vi "Dashboard Main.vi"() -> ()   [LabVIEW 2013]
uses:
  Vision/TargetType.ctl
  <vilib>/event_ctls.llb/eventvkey.ctl
  <vilib>/Rock Robotics/WPI/Dashboard/WPI_DashboardLogging Global.vi
  <vilib>/Utility/config.llb/Write Key (String).vi
  <vilib>/Utility/config.llb/Write Key (I32).vi
  <vilib>/Utility/config.llb/NI_LVConfig.lvlib
panel:
  out "Image Message":string="Timeout in Camera Communications"
  in  "Rec Mode":enum32{"Stop", "Record", "Playback"}(radio)
  in  "Dashboard Tab":T1(tab)
  in  "Camera Settings":T2={"Frame Rate"=30, "Compression"=30, "Size"=1} {"Frame Rate" scale=1.0..30.0; "Size" items=["640x480", "320x240", "160x120"]}
  out "MotorSliders R":cluster{"MotorSlide1":dbl, "MotorSlide2":dbl} {"MotorSlide2" scale=-1.0..1.0 scale format="%#_2e"; "MotorSlide1" scale=-1.0..1.0 scale format="%#_2e"}
  out "MotorChart R":cluster{"Numeric":dbl, "Numeric":dbl}(graph)
  out "MotorSliders L":T3 {"MotorSlide4 2" scale=0.0..14.0 scale format="%#_2e"; "MotorSlide2" scale=-1.0..1.0 scale format="%#_2e"; "MotorSlide1" scale=-1.0..1.0 scale format="%#_2e"}
  out "MotorChart L":T4(graph)
  out "JS1 Z":dbl(slide) scale=-1.0..1.0 scale format="%#_2e"
  out "Joystick 1":cluster{"X":dbl, "Y":dbl}[](graph)
  out "JS Buttons 1":T5
  out "JS2 Z":dbl(slide) scale=-1.0..1.0 scale format="%#_2e"
  out "Joystick 2":cluster{"X":dbl, "Y":dbl}[](graph)
  out "JS Buttons 2":T5
  out "Mode":T6(ring)=enum."Auto Disabled"
  out "Camera IP":string
  in  "DB Camera Config":bool
  out "fps":dbl format="%#.1g"
  out "Mbps":dbl format="%#.1g"
  out "Mbps 2":bool
  out "LED 1":bool
  in  "Color Components":T7={"Hue"={110.0, 142.0}, "Sat"={138.0, 255.0}, "Val"={139.0, 198.0}} {"Val" scale=0.0..255.0; "Sat" scale=0.0..255.0; "Hue" scale=0.0..255.0 scale format="%#_3g"}
  out "Distances":T9(array[cluster])
  in  "Test Slider":dbl(slide) scale=0.0..100.0 scale format="%#_3g"
  in  "On/Off":bool caption="Solenoid"
  in  "Test Name":u16(ring) items=["Select the test to run...", "Example Test", "-------------------------------", "List of tests is built in robot code.", "Replace with your own automated tests."]
  in  "Test Tree":string(tree)
  in  "Motor":cluster{"Value":dbl, "Enable":bool} {"Value" scale=-1.0..1.0 scale format="%#_3g"}
  out "Progress":T10 {"Test Progress" scale=0.0..100.0}
  in  "Rev/Fwd":cluster{"Forward":bool, "Reverse":bool}
  in  "Test Ring":u16(ring) items=["Auto", "Fixed indoor", "Fixed outdoor 1", "Fixed outdoor 2", "Fixed fluorescent 1", "Fixed fluorescent 2", "Hold current"]
  in  "Listbox":i32(listbox)
  out "Tree":string(tree)
  out "Camera Image":T11(plugin-control)
  in  "Enable":bool
  # "Left"
  # "Front"
  # "Right"
  # "Battery"
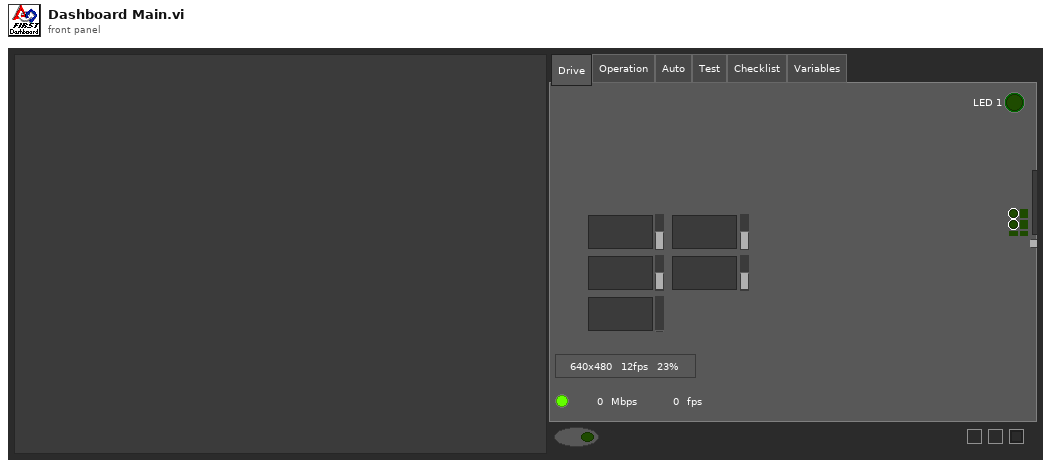
[diagram p1: front panel]
types:
  T1 = enum32{"Drive", "Operation", "Auto", "Test", "Checklist", "Variables"}
  T2 = cluster{"Frame Rate":i32, "Compression":i32, "Size":u16}
  T3 = cluster{"MotorSlide1":dbl, "MotorSlide2":dbl, "MotorSlide4 2":dbl}
  T4 = cluster{"Numeric":dbl, "Numeric":dbl, "Battery":sgl}
  T5 = cluster{bool, bool, bool, bool, bool, bool, bool, bool, bool, bool, bool, bool}
  T6 = enum8{"Tele-Op Disabled", "Tele-Op Enabled", "Auto Disabled", "Auto Enabled", "Test Disabled", "Test Enabled", ""}
  T7 = cluster{"Hue":cluster{dbl, dbl}, "Sat":cluster{dbl, dbl}, "Val":cluster{dbl, dbl}}
  T8 = typedef "TargetType.ctl" = enum16{"Not Hot", "Hot"}
  T9 = cluster{"Distance (ft)":dbl, "Target Center (-1 to 1)":cluster{"X":dbl, "Y":dbl}, "Left":bool, "State":T8}[]
  T10 = cluster{"Test Progress":u8, "Test Progress Text":string}
  T11 = typedef "IMAQ Image.ctl" = refnum<image>
  T12 = typedef "Image Type" = u32
  T13 = cluster{cluster{dbl, dbl}, cluster{dbl, dbl}, cluster{dbl, dbl}}
  T14 = cluster{"Digital Inputs":bool[], "Digital Outputs":bool[]}
  T15 = cluster{"Competition mode":bool, "Robot Link":bool, "Autonomous":bool, "Enabled":bool, "E-Stop":bool, "Simulated":bool, "TestMode":bool, "Docked Window":bool}
  T16 = typedef "NI_LVConfig.lvlib/Config Data RefNum.ctl" = refnum<k1>
  T17 = typedef "eventvkey.ctl" = enum16{"ASCII", "Enter", "Return", "Shift", "Ctrl", "Alt", "Cmd", "Opt", "Caps", "NumLock", "Clear", "Break", "Up", "Down", "Left", "Right", "Insert", "Delete", "Home", "End", "PageUp", "PageDown", "Escape", "Help", "Pause", "ScrollLock", "F1", "F2", "F3", "F4", "F5", "F6", "F7", "F8", "F9", "F10", "F11", "F12", "F13", "F14", "F15", "F16", "F17", "F18", "F19", "F20", "F21", "F22", "F23", "F24", "Play", "VolumeUp", "VolumeDown", "Mute", "Two Byte Char"}
  T18 = cluster{"Image Size":bool, "Image Type":bool, "Pixel Value":bool, "ROI Information":bool, "Zoom Factor":bool}
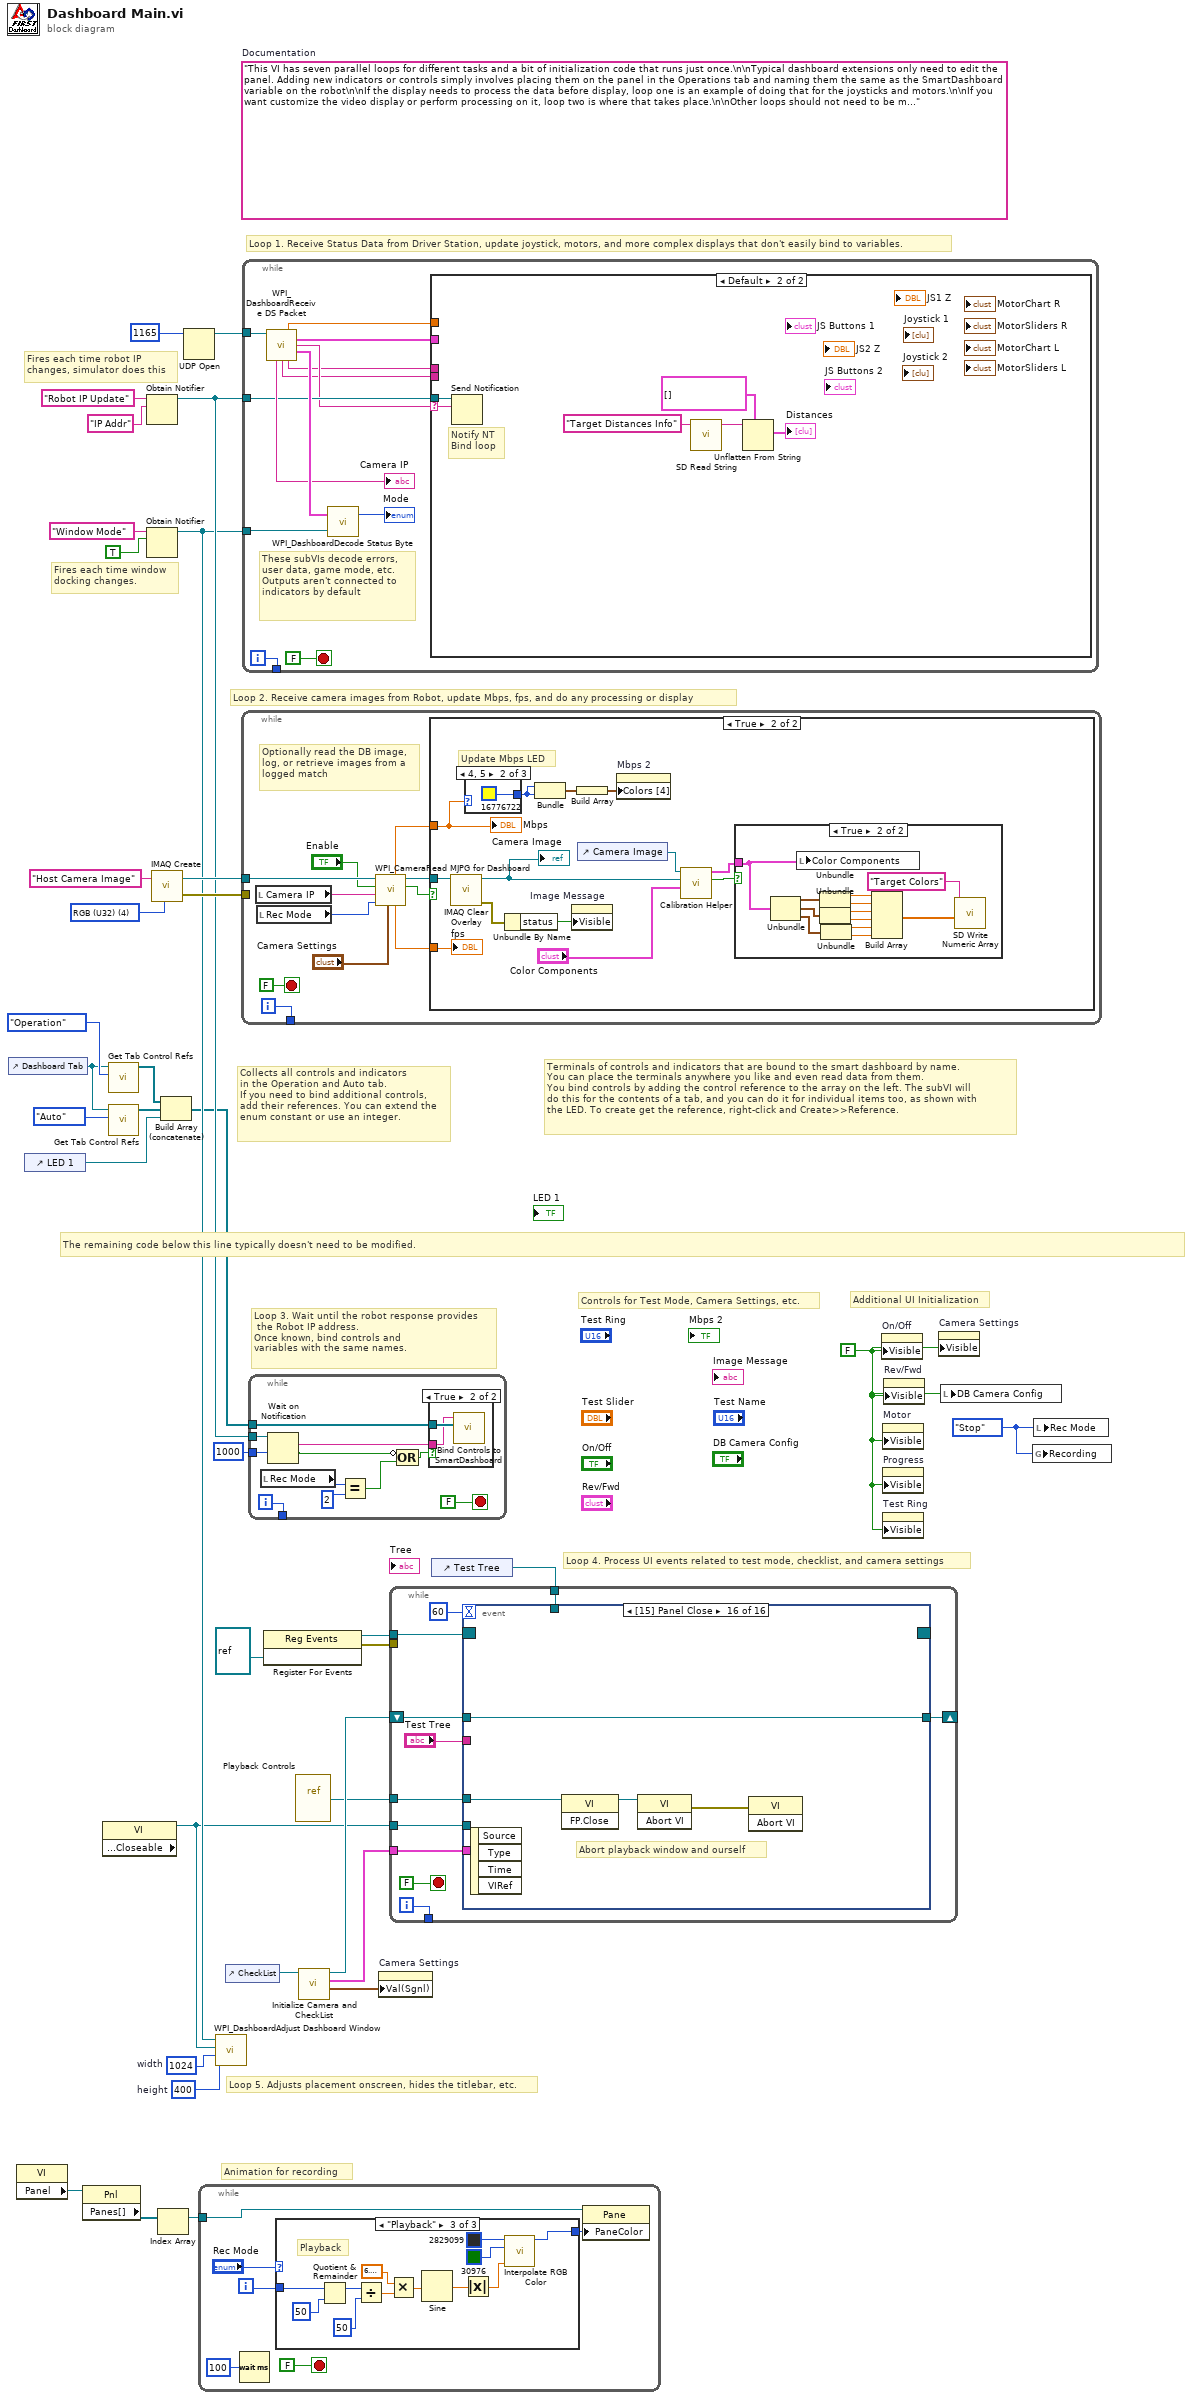
[diagram p0: block diagram]
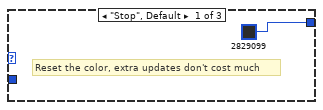
[diagram p2: hidden frame]
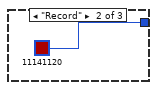
[diagram p3: hidden frame]
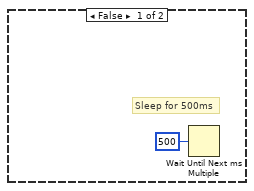
[diagram p5: hidden frame]
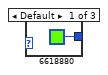
[diagram p7: hidden frame]
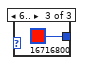
[diagram p8: hidden frame]
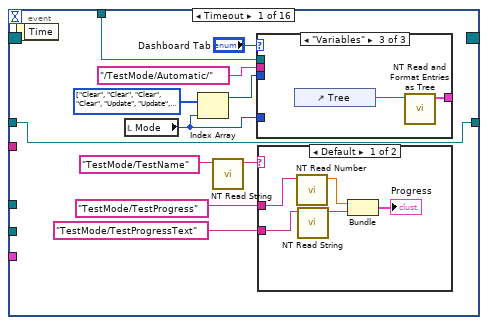
[diagram p9: hidden frame]
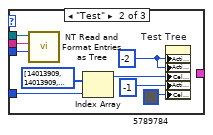
[diagram p11: hidden frame]
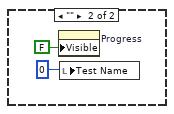
[diagram p12: hidden frame]
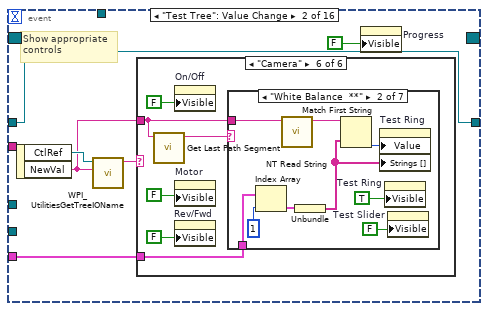
[diagram p13: hidden frame]
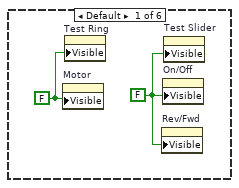
[diagram p14: hidden frame]
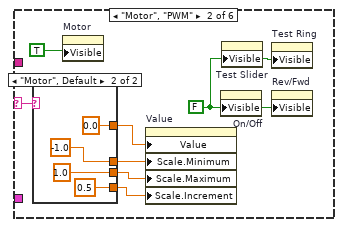
[diagram p15: hidden frame]
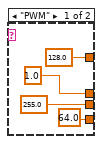
[diagram p16: hidden frame]
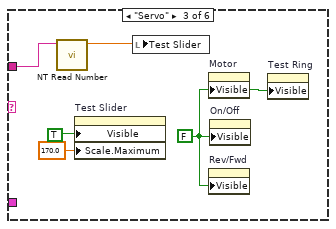
[diagram p17: hidden frame]
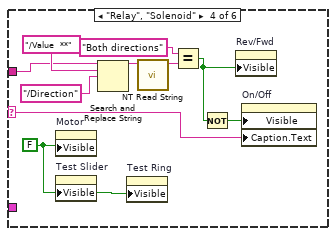
[diagram p18: hidden frame]
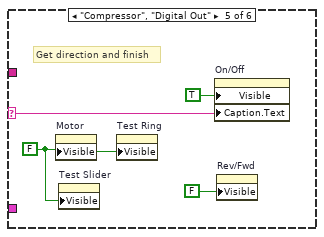
[diagram p19: hidden frame]
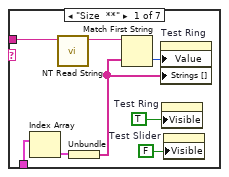
[diagram p20: hidden frame]
diagram:
  w8 = enum32{"Stop", "Record", "Playback"}."Stop" ("Rec Mode")
  w11 = 400  # height
  w12 = 1024  # width
  w25 = FALSE ("Visible")
  (unwired) "This VI has seven parallel loops for different tasks and a bit of initialization code that runs just once.\n\nTypical dashboard extensions only need to edit the panel. Adding new indicators or controls simply involves placing them on the panel in the Operations tab and naming them the same as the SmartDashboard variable on the robot\n\nIf the display needs to process the data before display, loop one is an example of doing that for the joysticks and motors.\n\nIf you want customize the video display or perform processing on it, loop two is where that takes place.\n\nOther loops should not need to be modified. They are pretty standard, and document the task they perform."  # Documentation
  w35 = T12 4 items=["Grayscale (U8)", "Grayscale (I16)", "Grayscale (SGL)", "Complex (CSG)", "RGB (U32)", "HSL (U32)", "RGB (U64)"] ("Image Type")
  # "Controls for Test Mode, Camera Settings, etc."
  # "Additional UI Initialization"
  # "Animation for recording"
  # "Fires each time robot IP\nchanges, simulator does this"
  # "Fires each time window\ndocking changes."
  # "Collects all controls and indicators\nin the Operation and Auto tab.\nIf you need to bind additional controls,\nadd their references. You can extend the\nenum constant or use an integer."
  # "The remaining code below this line typically doesn't need to be modified."
  # "Loop 4. Process UI events related to test mode, checklist, and camera settings"
  # "Terminals of controls and indicators that are bound to the smart dashboard by name.\nYou can place the terminals anywhere you like and even read data from them.\nYou bind controls by adding the control reference to the array on the left. The subVI will\ndo this for the contents of a tab, and you can do it for individual items too, as shown with\nthe LED. To create get the reference, right-click and Create>>Reference."
  # "Loop 3. Wait until the robot response provides\n the Robot IP address.\nOnce known, bind controls and\nvariables with the same names."
  # "Loop 5. Adjusts placement onscreen, hides the titlebar, etc."
  # "Loop 1. Receive Status Data from Driver Station, update joystick, motors, and more complex displays that don't easily bind to variables."
  # "Loop 2. Receive camera images from Robot, update Mbps, fps, and do any processing or display"
  n1 = control-ref of="Dashboard Tab"() -> (w6:refnum<vi>)
  n2 = property class="VI"() -> ("Panel"=w19:refnum<vi>)  [unwired: 2 in, 2 out]
  n3 = control-ref of="LED 1"() -> (w1:refnum<vi>)
  n4 = property class="Pnl"(reference=w19) -> ("Panes[]"=w20:refnum<vi>[])  [unwired: 1 in, 2 out]
  n5 = property class="VI" props=["Front Panel.Closeable"]() -> (reference out=w7:refnum<vi>)  [unwired: 2 in, 2 out]
  n6 = call <vilib>:"Get Tab Control Refs.vi"("Page Index"=T1."Operation" ("Dashboard Tab"), "TabControl in"=w6) -> ("ControlsOnPage"=w4:refnum<vi>[])  [unwired: 9 in]
  n7 = call <vilib>:"Get Tab Control Refs.vi"("Page Index"=T1."Auto" ("Dashboard Tab"), "TabControl in"=w6) -> ("ControlsOnPage"=w5:refnum<vi>[])  [unwired: 9 in]
  n8 = Obtain Notifier(name (unnamed)="Robot IP Update", notification data type="IP Addr" ("name (unnamed)")) -> (notifier out=w29:refnum<notifier>)  [unwired: 2 in, 2 out]
  n9 = Obtain Notifier(name (unnamed)="Window Mode", notification data type=TRUE) -> (notifier out=w10:refnum<notifier>)  [unwired: 2 in, 2 out]
  n10 = call "IMAQ Create"("Image Name"="Host Camera Image", "Image Type"=w35) -> ("New Image"=w33:T11, "error out"=w32:errorcluster)  [unwired: 2 in, 1 out]
  n11 = Index Array(array=w20) -> (element=w18:refnum<vi>)  [unwired: 1 in]
  n12 = Build Array (concatenate)(w4, w5, w1) -> (w3:refnum<vi>[])
  n13 = UDP Open(11:u16 1165 ("port")) -> (port=w36:refnum<k16>)  [unwired: 2 in, 4 out]
  n14 = while {
    tunnel: w18 -> [w39]
    i -> [w42]
    stop <- FALSE stop-if-true
    n15 = Wait (ms)(milliseconds to wait=u32 100) -> ()  [unwired: 1 out]
    n16 = case shown="\"Playback\"" "Rec Mode" {
      tunnel: w42 -> [_ _ w57]
      tunnel: [u32 2829099 ("Base Color") u32 11141120 ("Target Color") w46] -> w38
      frame "Stop", Default {
        # "Reset the color, extra updates don't cost much"
      }
      frame "Record" {
      }
      frame "Playback" {
        # "Playback"
        n17 = Quotient & Remainder(x=w57, y=u32 50 ("milliseconds to wait")) -> (x-y*floor(x/y)=w53:u32)  [unwired: 1 out]
        n18 = Divide(x=w53, y=u32 50 ("milliseconds to wait")) -> (x/y=w50:dbl)
        n19 = Multiply(x=6.283185307179586, y=w50) -> (x*y=w55:dbl)
        n20 = Sine(x=w55) -> (sin(x)=w54:dbl)
        n21 = Absolute Value(x=w54) -> (abs(x)=w47:dbl)
        n22 = call "Interpolate RGB Color.vi"("Proportion"=w47, "Target Color"=u32 30976, "Base Color"=u32 2829099) -> ("Result Color"=w46:u32)  [unwired: 8 in]
      }
    }
    n23 = property class="Pane"(reference=w39, "PaneColor"=w38) -> ()  [unwired: 1 in, 2 out]
  }
  n24 = call <vilib>:"WPI_DashboardAdjust Dashboard Window.vi"("height"=w11, "width"=w12, "reference in"=w7, "Notifier in"=w10) -> ()  [unwired: 8 in]
  n25 = control-ref of="CheckList"() -> (w9:refnum<vi>)
  n26 = while {
    tunnel: w33 -> [w66]
    tunnel: w32 -> [_]
    tunnel: [w67] -> _
    i -> [w67]
    stop <- FALSE stop-if-true
    # "Optionally read the DB image,\nlog, or retrieve images from a\nlogged match"
    n27 = local read "Camera IP"() -> (w59:string)
    n28 = local read "Rec Mode"() -> (w58:enum32{"Stop", "Record", "Playback"})
    n29 = call <vilib>:"WPI_CameraRead MJPG for Dashboard.vi"("Camera Settings"="Camera Settings", "Rec Mode"=w58, "Camera IP"=w59, "Enable"="Enable", "Refnum in"=w66) -> ("Active"=w63:bool, "Refnum out"=w65:T11, "FPS"=w62:dbl, "Bandwidth (Mbps)"=w61:dbl)  [unwired: 3 in]
    n30 = case shown="True" w63 {
      tunnel: w65 -> [_ w77]
      tunnel: w61 -> [_ w76]
      tunnel: w62 -> [_ w75]
      frame False {
        # "Sleep for 500ms"
        n31 = Wait Until Next ms Multiple(millisecond multiple=u32 500) -> ()  [unwired: 1 out]
      }
      frame True {
        # "Update Mbps LED"
        n32 = call "IMAQ Clear Overlay"("Image"=w77) -> ("error out"=w81:errorcluster, "Image Out"=w74:T11)  [unwired: 2 in, 7 out]
        "Camera Image" <- w74
        n33 = case shown="4, 5" w76 {
          tunnel: [u32 6618880 ("Color Box") u32 16776722 ("Color Box") u32 16716800 ("Color Box")] -> w78
          frame Default {
          }
          frame 4, 5 {
          }
          frame 6.. {
          }
        }
        n34 = Unbundle By Name(w81) -> ("status"=w82:bool)
        n35 = Bundle("Color Box"=w78, "Color Box"=w78) -> (w80:cluster{"Color Box":u32, "Color Box":u32})  [unwired: 1 out]
        n36 = property on="Image Message" class="Str"("Visible"=w82) -> ()  [unwired: 2 in, 2 out]
        n37 = Build Array(w80) -> (w79:cluster{"Color Box":u32, "Color Box":u32}[])
        n38 = control-ref of="Camera Image"() -> (w70:refnum<vi>)
        n39 = property on="Mbps 2" class="Bool (strict)"("Colors [4]"=w79) -> ()  [unwired: 2 in, 2 out]
        n40 = call "Calibration Helper.vi"("Color Components"="Color Components", "Image"=w74, "Image Ctl Refnum"=w70) -> ("Changed"=w72:bool, "output color"=w71:T13)  [unwired: 7 in]
        n41 = case shown="True" w72 {
          tunnel: w71 -> [_ w94]
          frame False {
          }
          frame True {
            n42 = Unbundle(w94) -> (w93:cluster{dbl, dbl}, w92:cluster{dbl, dbl}, w91:cluster{dbl, dbl})
            n43 = local write "Color Components"(w94) -> ()
            n44 = Unbundle(w93) -> (w90:dbl, w89:dbl)
            n45 = Unbundle(w92) -> (w88:dbl, w87:dbl)
            n46 = Unbundle(w91) -> (w86:dbl, w85:dbl)
            n47 = Build Array(w90, w89, w88, w87, w86, w85) -> (w84:dbl[])
            n48 = call <vilib>:"SD Write Numeric Array.vi"("Numeric Array"=w84, "Name"="Target Colors") -> ()  [unwired: 8 in, 2 out]
          }
        }
        "Mbps" <- w76
        "fps" <- w75
      }
    }
  }
  n49 = while {
    tunnel: w36 -> [w108]
    tunnel: w29 -> [w103]
    tunnel: w10 -> [w107]
    tunnel: [w104] -> _
    i -> [w104]
    stop <- FALSE stop-if-true
    # "These subVIs decode errors, user data, game mode, etc.\nOutputs aren't connected to indicators by default"
    n50 = call <vilib>:"WPI_DashboardReceive DS Packet.vi"("Recv Socket"=w108) -> ("Battery"=w98:sgl, "Driver Station"=w99:T14, "Robot IP Address"=w102:string, "Status"=w109:T15, "Camera IP Address"=→"Camera IP":string, "Low Priority User Data"=w101:string, "High Priority User Data"=w100:string)  [unwired: 1 in, 7 out]
    n51 = call <vilib>:"WPI_DashboardDecode Status Byte.vi"("Window Mode Notifier"=w107, "Status"=w109) -> ("Mode"=→"Mode":T6)  [unwired: 1 out]
    n52 = case shown="Default" w102 {
      selector: w102 -> [_ w115]
      tunnel: w103 -> [_ w116]
      tunnel: w101 -> [_ _]
      tunnel: w100 -> [_ _]
      tunnel: w99 -> [_ _]
      tunnel: w98 -> [_ _]
      frame "0.0.0.0" {
        # "DS not sending packets, or no robot exists yet.\nDon't poll the variables"
      }
      frame Default {
        # "Notify NT\nBind loop"
        n53 = Send Notification(notification=w115, notifier=w116) -> ()  [unwired: 1 in, 2 out]
        n54 = call <vilib>:"SD Read String.vi"("Name"="Target Distances Info") -> ("String"=w114:string)  [unwired: 8 in, 2 out]
        n55 = Unflatten From String(type=T9 [] ("Distances"), binary string=w114) -> (value=→"Distances":T9)  [unwired: 3 in, 2 out]
      }
    }
  }
  n56 = while {
    tunnel: w3 -> [w127]
    tunnel: w29 -> [w125]
    tunnel: [w123] -> _
    tunnel: u32 1000 ("milliseconds to wait") -> [w122]
    i -> [w123]
    stop <- FALSE stop-if-true
    n57 = local read "Rec Mode"() -> (w118:enum32{"Stop", "Record", "Playback"})
    n58 = Wait on Notification(notifier=w125, timeout in ms (-1)=w122) -> (notification=w124:string, timed out?=w120:bool)  [unwired: 2 in, 2 out]
    n59 = Equal?(x=w118, y=u16 2 ("Rec Mode")) -> (x = y?=w119:bool)
    n60 = Compound Arithmetic op=OR(invert w120, w119) -> (w121:bool)
    n61 = case shown="True" w121 {
      tunnel: w127 -> [_ w129]
      tunnel: w124 -> [_ w128]
      frame False {
      }
      frame True {
        n62 = call <vilib>:"Bind Controls to SmartDashboard.vi"("Bound Control Refs"=w129, "Server IP Address"=w128) -> ()  [unwired: 10 in]
      }
    }
  }
  n63 = register-events(refnum<vi> refnum) -> (reference out=w16:refnum<event-registration>, error out=w15:errorcluster)  [unwired: 2 in]
  n64 = vi-ref "Playback Controls.vi"() -> (w17:refnum<vi>)
  n65 = call "Initialize Camera and CheckList.vi"("ListBox in"=w9) -> ("Cluster"=w23:cluster{"value":i32, "value":i32, "index":i32}, "Array"=w24:cluster{string[]}[], "File Refnum"=w22:T16)  [unwired: 8 in]
  n66 = property on="Camera Settings" class="Clust (strict)"("Val(Sgnl)"=w23) -> ()  [unwired: 2 in, 2 out]
  n67 = control-ref of="Test Tree"() -> (w21:refnum<vi>)
  n68 = while {
    tunnel: w24 -> [w137]
    shift-right: [w136] -> _
    shift-left: w22 -> [w135]
    tunnel: [w134] -> _
    tunnel: w21 -> [w133]
    tunnel: w17 -> [w132]
    tunnel: w16 -> [w131]
    tunnel: w15 -> [_]
    tunnel: w7 -> [w130]
    i -> [w134]
    stop <- FALSE stop-if-true
    n69 = event shown="[15] Panel Close" {
      selector: w131 -> [_ _ _ _ _ _ _ _ _ _ _ _ _ _ _ _]
      dyn-events: [_ _ _ _ _ _ _ _ _ _ _ _ _ w375 _ _] -> _
      timeout: u32 60 ("milliseconds to wait") -> [_ _ _ _ _ _ _ _ _ _ _ _ _ _ _ _]
      tunnel: w133 -> [w147 _ _ _ _ _ _ _ _ _ _ _ _ _ _ _]
      tunnel: "Test Tree" -> [_ _ _ _ _ _ _ _ w344 w352 w354 w358 w366 _ _ _]
      tunnel: w137 -> [_ w171 _ _ _ _ w308 w338 _ _ _ _ _ _ _ _]
      tunnel: [w141 w170 w269 w274 w282 w294 w307 w331 w343 w350 w353 w357 w365 w377 w391 w392] -> w136
      tunnel: w135 -> [w141 w170 w269 w274 w282 w294 w306 w331 w343 w350 w353 w357 w365 w377 w391 w392]
      tunnel: w132 -> [_ _ _ _ _ _ _ _ _ _ _ _ _ w378 _ w395]
      tunnel: w130 -> [_ _ _ _ _ _ _ _ _ _ _ _ _ w373 _ _]
      event Timeout {
        w146 = enum16{"Update", "Clear"}[] [enum."Clear", enum."Clear", enum."Clear", enum."Clear", enum."Update", enum."Update", enum."Clear"] items=["Update", "Clear"]
        n70 = event-data() -> ()  [unwired: 1 in, 1 out]
        n71 = local read "Mode"() -> (w144:T6)
        n72 = Index Array(array=w146, index=w144) -> (element=w145:enum16{"Update", "Clear"})
        n73 = call <vilib>:"NT Read String.vi"("Name"="TestMode/TestName") -> ("String"=w150:string)  [unwired: 9 in, 1 out]
        n74 = case shown="\"Variables\"" "Dashboard Tab" {
          tunnel: w147 -> [_ w160 _]
          tunnel: "/TestMode/Automatic/" ("Name Pattern") -> [_ w159 _]
          tunnel: w145 -> [_ w158 _]
          tunnel: w144 -> [_ w156 _]
          tunnel: [_ _ w162] -> _
          frame "Operation", Default {
          }
          frame "Test" {
            w155 = -2 ("Active Item:Row Number")
            n75 = call <vilib>:"NT Read and Format Entries as Tree.vi"("Operation"=w158, "Name Pattern"=w159, "Tree Refnum"=w160) -> ()  [unwired: 7 in, 2 out]
            n76 = Index Array(array=u32[] [14013909, 14013909, 14013909, 14013909, 14013909, 16777215, 14013909], index=w156) -> (element=w154:u32)
            n77 = property on="Test Tree" class="Tree (strict)"("Active Item Row Number"=w155, "ActiveColNum"=w155, "CellBG"=w154, "Active Item Row Number"=-1 ("Active Item:Row Number"), "CellBG"=u32 5789784 ("Color Box")) -> ()  [unwired: 2 in, 2 out]
          }
          frame "Variables" {
            n78 = control-ref of="Tree"() -> (w161:refnum<vi>)
            n79 = call <vilib>:"NT Read and Format Entries as Tree.vi"("Tree Refnum"=w161) -> ("Formatted Strings"=w162:cluster{"Name":string, "Value":string}[])  [unwired: 9 in, 1 out]
          }
        }
        n80 = case shown="Default" w150 {
          tunnel: "TestMode/TestProgress" ("Name") -> [w164 _]
          tunnel: "TestMode/TestProgressText" ("Name") -> [w163 _]
          frame Default {
            n81 = call <vilib>:"NT Read Number.vi"("Name"=w164) -> ("Numeric"=w165:dbl)  [unwired: 9 in, 1 out]
            n82 = call <vilib>:"NT Read String.vi"("Name"=w163) -> ("String"=w166:string)  [unwired: 9 in, 1 out]
            n83 = Bundle("Numeric"=w165, "String"=w166) -> (→"Progress":cluster{"Numeric":dbl, "String":string})  [unwired: 1 in]
          }
          frame "" {
            n84 = property on="Progress" class="Clust (strict)"("Visible"=FALSE) -> ()  [unwired: 2 in, 2 out]
            n85 = local write "Test Name"(u16 0) -> ()
          }
        }
      }
      event "Test Tree": Value Change {
        # "Show appropriate\ncontrols"
        n86 = event-data() -> ("CtlRef"=w174:refnum<vi>, "NewVal"=w172:string)  [unwired: 1 in]
        n87 = call <vilib>:"WPI_UtilitiesGetTreeIOName.vi"("NewVal"=w172, "TreeControl in"=w174) -> ("I/O Name"=w175:string)  [unwired: 9 in]
        n88 = case shown="\"Camera\"" w175 {
          selector: w175 -> [_ w182 _ w200 w209 _]
          tunnel: w172 -> [_ _ w197 w199 _ w216]
          tunnel: w171 -> [_ _ _ _ _ w215]
          frame Default {
            w177 = FALSE ("Visible")
            w176 = FALSE ("Visible")
            n89 = property on="Motor" class="Clust (strict)"("Visible"=w176) -> ()  [unwired: 2 in, 2 out]
            n90 = property on="Test Ring" class="Ring (strict)"("Visible"=w176) -> ()  [unwired: 2 in, 2 out]
            n91 = property on="Rev/Fwd" class="Clust (strict)"("Visible"=w177) -> ()  [unwired: 2 in, 2 out]
            n92 = property on="On/Off" class="Bool (strict)"("Visible"=w177) -> ()  [unwired: 2 in, 2 out]
            n93 = property on="Test Slider" class="Slide (strict)"("Visible"=w177) -> ()  [unwired: 2 in, 2 out]
          }
          frame "Motor", "PWM" {
            w183 = FALSE ("Visible")
            n94 = case shown="\"Motor\", Default" w182 {
              tunnel: [1.0 ("Value") -1.0 ("Value")] -> w181
              tunnel: [255.0 ("Value") 1.0 ("Value")] -> w180
              tunnel: [128.0 ("Value") 0.0 ("Value")] -> w179
              tunnel: [64.0 ("Value") 0.5 ("Value")] -> w178
              frame "PWM" {
              }
              frame "Motor", Default {
              }
            }
            n95 = property on="Motor" class="Clust (strict)"("Visible"=TRUE) -> ()  [unwired: 2 in, 2 out]
            n96 = property on="Value" class="Slide (strict)"("Value"=w179, "Scale.Minimum"=w181, "Scale.Maximum"=w180, "Scale.Increment"=w178) -> ()  [unwired: 2 in, 2 out]
            n97 = property on="On/Off" class="Bool (strict)"("Visible"=w183) -> ()  [unwired: 2 in, 2 out]
            n98 = property on="Test Slider" class="Slide (strict)"("Visible"=w183) -> ()  [unwired: 2 in, 2 out]
            n99 = property on="Test Ring" class="Ring (strict)"("Visible"=w183) -> ()  [unwired: 2 in, 2 out]
            n100 = property on="Rev/Fwd" class="Clust (strict)"("Visible"=w183) -> ()  [unwired: 2 in, 2 out]
          }
          frame "Servo" {
            w195 = FALSE ("Visible")
            n101 = call <vilib>:"NT Read Number.vi"("Name"=w197) -> ("Numeric"=w196:dbl)  [unwired: 9 in, 1 out]
            n102 = property on="Test Slider" class="Slide (strict)"("Visible"=TRUE, "Scale.Maximum"=170.0 ("Scale.Range:Maximum")) -> ()  [unwired: 2 in, 2 out]
            n103 = local write "Test Slider"(w196) -> ()
            n104 = property on="Motor" class="Clust (strict)"("Visible"=w195) -> ()  [unwired: 2 in, 2 out]
            n105 = property on="Rev/Fwd" class="Clust (strict)"("Visible"=w195) -> ()  [unwired: 2 in, 2 out]
            n106 = property on="On/Off" class="Bool (strict)"("Visible"=w195) -> ()  [unwired: 2 in, 2 out]
            n107 = property on="Test Ring" class="Ring (strict)"("Visible"=w195) -> ()  [unwired: 2 in, 2 out]
          }
          frame "Relay", "Solenoid" {
            w198 = FALSE ("Visible")
            n108 = property on="Motor" class="Clust (strict)"("Visible"=w198) -> ()  [unwired: 2 in, 2 out]
            n109 = property on="Test Slider" class="Slide (strict)"("Visible"=w198) -> ()  [unwired: 2 in, 2 out]
            n110 = Search and Replace String(input string=w199, search string="/Value  **", replace string="/Direction") -> (result string=w205:string)  [unwired: 5 in, 3 out]
            n111 = property on="Test Ring" class="Ring (strict)"("Visible"=w198) -> ()  [unwired: 2 in, 2 out]
            n112 = call <vilib>:"NT Read String.vi"("Name"=w205) -> ("String"=w203:string)  [unwired: 9 in, 1 out]
            n113 = Equal?(x="Both directions", y=w203) -> (x = y?=w201:bool)
            n114 = Not(x=w201) -> (.not. x?=w202:bool)
            n115 = property on="Rev/Fwd" class="Clust (strict)"("Visible"=w201) -> ()  [unwired: 2 in, 2 out]
            n116 = property on="On/Off" class="Bool (strict)"("Visible"=w202, "Caption.Text"=w200) -> ()  [unwired: 2 in, 2 out]
          }
          frame "Compressor", "Digital Out" {
            w208 = FALSE ("Visible")
            # "Get direction and finish"
            n117 = property on="Motor" class="Clust (strict)"("Visible"=w208) -> ()  [unwired: 2 in, 2 out]
            n118 = property on="Test Slider" class="Slide (strict)"("Visible"=w208) -> ()  [unwired: 2 in, 2 out]
            n119 = property on="Test Ring" class="Ring (strict)"("Visible"=w208) -> ()  [unwired: 2 in, 2 out]
            n120 = property on="On/Off" class="Bool (strict)"("Visible"=TRUE, "Caption.Text"=w209) -> ()  [unwired: 2 in, 2 out]
            n121 = property on="Rev/Fwd" class="Clust (strict)"("Visible"=FALSE) -> ()  [unwired: 2 in, 2 out]
          }
          frame "Camera" {
            n122 = call <vilib>:"Get Last Path Segment.vi"("String in"=w216) -> ("String out"=w217:string)  [unwired: 10 in]
            n123 = property on="On/Off" class="Bool (strict)"("Visible"=FALSE) -> ()  [unwired: 2 in, 2 out]
            n124 = property on="Motor" class="Clust (strict)"("Visible"=FALSE) -> ()  [unwired: 2 in, 2 out]
            n125 = property on="Rev/Fwd" class="Clust (strict)"("Visible"=FALSE) -> ()  [unwired: 2 in, 2 out]
            n126 = case shown="\"White Balance  **\"" w217 {
              tunnel: w216 -> [w223 w232 w241 w250 w259 _ w265]
              tunnel: w215 -> [w221 w229 w238 w247 w256 _ _]
              frame "Size  **" {
                n127 = Index Array(array=w221) -> (element=w220:cluster{string[]})  [unwired: 1 in]
                n128 = call <vilib>:"NT Read String.vi"("Name"=w223) -> ("String"=w222:string)  [unwired: 9 in, 1 out]
                n129 = Unbundle(w220) -> (w218:string[])
                n130 = Match First String(2:w218, 3:w222) -> (0:w219:i32)  [unwired: 1 out]
                n131 = property on="Test Ring" class="Ring (strict)"("Value"=w219, "Strings []"=w218) -> ()  [unwired: 2 in, 2 out]
                n132 = property on="Test Ring" class="Ring (strict)"("Visible"=TRUE) -> ()  [unwired: 2 in, 2 out]
                n133 = property on="Test Slider" class="Slide (strict)"("Visible"=FALSE) -> ()  [unwired: 2 in, 2 out]
              }
              frame "White Balance  **" {
                n134 = Index Array(array=w229, index=1) -> (element=w230:cluster{string[]})
                n135 = call <vilib>:"NT Read String.vi"("Name"=w232) -> ("String"=w231:string)  [unwired: 9 in, 1 out]
                n136 = Unbundle(w230) -> (w227:string[])
                n137 = Match First String(2:w227, 3:w231) -> (0:w226:i32)  [unwired: 1 out]
                n138 = property on="Test Ring" class="Ring (strict)"("Value"=w226, "Strings []"=w227) -> ()  [unwired: 2 in, 2 out]
                n139 = property on="Test Ring" class="Ring (strict)"("Visible"=TRUE) -> ()  [unwired: 2 in, 2 out]
                n140 = property on="Test Slider" class="Slide (strict)"("Visible"=FALSE) -> ()  [unwired: 2 in, 2 out]
              }
              frame "Exposure  **" {
                n141 = Index Array(array=w238, index=2) -> (element=w239:cluster{string[]})
                n142 = call <vilib>:"NT Read String.vi"("Name"=w241) -> ("String"=w240:string)  [unwired: 9 in, 1 out]
                n143 = Unbundle(w239) -> (w235:string[])
                n144 = Match First String(2:w235, 3:w240) -> (0:w236:i32)  [unwired: 1 out]
                n145 = property on="Test Ring" class="Ring (strict)"("Value"=w236, "Strings []"=w235) -> ()  [unwired: 2 in, 2 out]
                n146 = property on="Test Ring" class="Ring (strict)"("Visible"=TRUE) -> ()  [unwired: 2 in, 2 out]
                n147 = property on="Test Slider" class="Slide (strict)"("Visible"=FALSE) -> ()  [unwired: 2 in, 2 out]
              }
              frame "Exposure Priority  **" {
                n148 = Index Array(array=w247, index=3) -> (element=w248:cluster{string[]})
                n149 = call <vilib>:"NT Read String.vi"("Name"=w250) -> ("String"=w249:string)  [unwired: 9 in, 1 out]
                n150 = Unbundle(w248) -> (w244:string[])
                n151 = Match First String(2:w244, 3:w249) -> (0:w245:i32)  [unwired: 1 out]
                n152 = property on="Test Ring" class="Ring (strict)"("Value"=w245, "Strings []"=w244) -> ()  [unwired: 2 in, 2 out]
                n153 = property on="Test Ring" class="Ring (strict)"("Visible"=TRUE) -> ()  [unwired: 2 in, 2 out]
                n154 = property on="Test Slider" class="Slide (strict)"("Visible"=FALSE) -> ()  [unwired: 2 in, 2 out]
              }
              frame "Color Enable  **" {
                n155 = Index Array(array=w256, index=4) -> (element=w257:cluster{string[]})
                n156 = call <vilib>:"NT Read String.vi"("Name"=w259) -> ("String"=w258:string)  [unwired: 9 in, 1 out]
                n157 = Unbundle(w257) -> (w253:string[])
                n158 = Match First String(2:w253, 3:w258) -> (0:w254:i32)  [unwired: 1 out]
                n159 = property on="Test Ring" class="Ring (strict)"("Value"=w254, "Strings []"=w253) -> ()  [unwired: 2 in, 2 out]
                n160 = property on="Test Ring" class="Ring (strict)"("Visible"=TRUE) -> ()  [unwired: 2 in, 2 out]
                n161 = property on="Test Slider" class="Slide (strict)"("Visible"=FALSE) -> ()  [unwired: 2 in, 2 out]
              }
              frame Default {
                n162 = property on="Test Ring" class="Ring (strict)"("Visible"=FALSE) -> ()  [unwired: 2 in, 2 out]
                n163 = property on="Test Slider" class="Slide (strict)"("Visible"=FALSE) -> ()  [unwired: 2 in, 2 out]
              }
              frame "Brightness  **", "Color Level  **", "Compression  **", "FPS  **", "Sharpness  **" {
                n164 = call <vilib>:"NT Read Number.vi"("Name"=w265) -> ("Numeric"=w264:dbl)  [unwired: 9 in, 1 out]
                n165 = local write "Test Slider"(w264) -> ()
                n166 = property on="Test Slider" class="Slide (strict)"("Visible"=TRUE, "Scale.Maximum"=100.0 ("Scale.Range:Maximum")) -> ()  [unwired: 2 in, 2 out]
                n167 = property on="Test Ring" class="Ring (strict)"("Visible"=FALSE) -> ()  [unwired: 2 in, 2 out]
              }
            }
          }
        }
        n168 = property on="Progress" class="Clust (strict)"("Visible"=FALSE) -> ()  [unwired: 2 in, 2 out]
      }
      event "Test Name": Mouse Enter {
        # "Populate the ring with the list of tests"
        n169 = event-data() -> ()  [unwired: 1 in, 1 out]
        n170 = call <vilib>:"NT Read String Array.vi"("Name"="TestMode/TestList") -> ("String Array"=w273:string[])  [unwired: 9 in, 1 out]
        n171 = Build Array (concatenate)("Select the test to run...", w273) -> (w272:string[])
        n172 = property on="Test Name" class="Ring (strict)"("Strings []"=w272) -> ()  [unwired: 2 in, 2 out]
      }
      event "Test Name": Value Change {
        w275 = FALSE ("Visible")
        # "Tell the robot the test name to run"
        n173 = event-data() -> ("NewVal"=w279:u16)  [unwired: 1 in]
        n174 = property on="Test Name" class="Ring (strict)"() -> ("Strings []"=w280:string[])  [unwired: 2 in, 2 out]
        n175 = local write "Progress"(T10 {"Test Progress"=0, "Test Progress Text"=""} ("Progress")) -> ()
        n176 = Index Array(array=w280, index=w279) -> (element=w278:string)
        n177 = call <vilib>:"NT Write String.vi"("String"=w278, "Name"="TestMode/TestName") -> ()  [unwired: 9 in, 1 out]
        n178 = property on="Progress" class="Clust (strict)"("Visible"=TRUE) -> ()  [unwired: 2 in, 2 out]
        n179 = property on="Motor" class="Clust (strict)"("Visible"=w275) -> ()  [unwired: 2 in, 2 out]
        n180 = property on="Test Slider" class="Slide (strict)"("Visible"=w275) -> ()  [unwired: 2 in, 2 out]
        n181 = property on="On/Off" class="Bool (strict)"("Visible"=w275) -> ()  [unwired: 2 in, 2 out]
        n182 = property on="Rev/Fwd" class="Clust (strict)"("Visible"=w275) -> ()  [unwired: 2 in, 2 out]
        n183 = property on="Test Ring" class="Ring (strict)"("Visible"=w275) -> ()  [unwired: 2 in, 2 out]
      }
      event "Listbox": Double Click {
        n184 = event-data() -> ("PlatMods.Shift"=w283:bool, "Row"=w285:i32)  [unwired: 1 in]
        n185 = case shown="True" w283 {
          tunnel: w285 -> [w289 _]
          tunnel: 1 -> [w288 _]
          frame False {
            n186 = property on="Listbox" class="LstBox (strict)"() -> ("Item Symbols"=w287:i32[])  [unwired: 2 in, 2 out]
            n187 = Replace Array Subset(array=w287, new element=w288, index=w289) -> (w286:i32[])
            n188 = property on="Listbox" class="LstBox (strict)"("Item Symbols"=w286) -> ()  [unwired: 2 in, 2 out]
          }
          frame True {
            w290 = 0 ("Top Row")
            n189 = property on="Listbox" class="LstBox (strict)"() -> ("Number of Rows"=w292:u32)  [unwired: 2 in, 2 out]
            n190 = Initialize Array(0, w292) -> (w291:i32[])
            n191 = property on="Listbox" class="LstBox (strict)"("Top Row"=w290, "Value"=w290, "Item Symbols"=w291) -> ()  [unwired: 2 in, 2 out]
          }
        }
      }
      event "Listbox": Key Down {
        n192 = event-data() -> ("VKey"=w296:T17)  [unwired: 1 in]
        n193 = case shown="\"Left\", \"Right\"" w296 {
          selector: w296 -> [w301 _]
          tunnel: eventvkey."Left" ("VKey") -> [w299 _]
          frame "Left", "Right" {
            n194 = Equal?(x=w299, y=w301) -> (x = y?=w300:bool)
            n195 = Select(t=0, s=w300, f=1) -> (s? t:f=w302:i32)
            n196 = property on="Listbox" class="LstBox (strict)"() -> ("Item Symbols"=w305:i32[])  [unwired: 2 in, 2 out]
            n197 = Replace Array Subset(array=w305, new element=w302, index="Listbox") -> (w304:i32[])
            n198 = property on="Listbox" class="LstBox (strict)"("Item Symbols"=w304) -> ()  [unwired: 2 in, 2 out]
          }
          frame Default {
          }
        }
      }
      event "DB Camera Config": Value Change {
        n199 = event-data() -> ("NewVal"=w309:bool)  [unwired: 1 in]
        n200 = case shown="False" w309 {
          tunnel: w308 -> [w318 _]
          tunnel: [w311 w329] -> w307
          tunnel: w306 -> [w310 w329]
          frame False {
            w325 = "Camera"
            w328 = FALSE ("Visible")
            n201 = local read "Camera Settings"() -> (w317:T2)
            n202 = Index Array(array=w318) -> (element=w321:cluster{string[]})  [unwired: 1 in]
            n203 = Unbundle(w317) -> ("Frame Rate"=w316:i32, "Compression"=w315:i32, "Size"=w319:u16)
            n204 = Unbundle(w321) -> (w320:string[])
            n205 = Index Array(array=w320, index=w319) -> (element=w314:string)
            n206 = call-poly <vilib>:"Write Key.vi"("section"=w325, "value"=w314, "key"="Size", "refnum"=w310) -> ("refnum out"=w327:T16)  [unwired: 2 in, 5 out]
            n207 = call-poly <vilib>:"Write Key.vi"("section"=w325, "value"=w316, "key"="FrameRate", "refnum"=w327) -> ("refnum out"=w326:T16)  [unwired: 1 in, 6 out]
            n208 = property on="Camera Settings" class="Clust (strict)"("Visible"=w328) -> ()  [unwired: 2 in, 2 out]
            n209 = local write "DB Camera Config"(w328) -> ()
            n210 = call-poly <vilib>:"Write Key.vi"("section"=w325, "value"=w315, "key"="Compression", "refnum"=w326) -> ("refnum out"=w312:T16)  [unwired: 1 in, 6 out]
            n211 = call <vilib>:"Close Config Data.vi"("refnum"=w312) -> ("file path"=w313:path)  [unwired: 2 in, 8 out]
            n212 = call <vilib>:"Open Config Data.vi"("configuration file path"=w313) -> ("refnum"=w311:T16)  [unwired: 8 in, 2 out]
          }
          frame True {
            n213 = property on="Camera Settings" class="Clust (strict)"("Visible"=TRUE) -> ()  [unwired: 2 in, 2 out]
          }
        }
      }
      event "Camera Settings": Value Change {
        n214 = event-data() -> ("NewVal"=w342:T2)  [unwired: 1 in]
        n215 = Index Array(array=w338) -> (element=w337:cluster{string[]})  [unwired: 1 in]
        n216 = Unbundle(w342) -> ("Frame Rate"=w333:i32, "Compression"=w332:i32, "Size"=w335:u16)
        n217 = Unbundle(w337) -> (w336:string[])
        n218 = Index Array(array=w336, index=w335) -> (element=w334:string)
        n219 = Format Into String(format string="%s   %dfps   %d%%", w334, w333, w332) -> (resulting string=w339:string)  [unwired: 2 in, 1 out]
        n220 = Build Array(w339) -> (w340:string[])
        n221 = property on="DB Camera Config" class="Bool (strict)"("Strings [4]"=w340) -> ()  [unwired: 2 in, 2 out]
      }
      event "Motor.Enable": Value Change {
        n222 = event-data() -> ("NewVal"=w348:bool)  [unwired: 1 in]
        n223 = Unbundle("Motor") -> ("Value"=w347:dbl)  [unwired: 1 out]
        n224 = Select(t=w347, s=w348, f=0.0) -> (s? t:f=w345:dbl)
        n225 = call <vilib>:"NT Write Number.vi"("Numeric"=w345, "Name"=w344) -> ()  [unwired: 9 in, 1 out]
      }
      event "Test Slider": Value Change {
        n226 = event-data() -> ("NewVal"=w351:dbl)  [unwired: 1 in]
        n227 = call <vilib>:"NT Write Number.vi"("Numeric"=w351, "Name"=w352) -> ()  [unwired: 9 in, 1 out]
      }
      event "On/Off": Value Change {
        n228 = event-data() -> ("NewVal"=w356:bool)  [unwired: 1 in]
        n229 = Boolean To (0,1)(Boolean=w356) -> (0, 1=w355:i16)
        n230 = call <vilib>:"NT Write Number.vi"("Numeric"=w355, "Name"=w354) -> ()  [unwired: 9 in, 1 out]
      }
      event "Rev/Fwd": Value Change {
        n231 = event-data() -> ("NewVal.Forward"=w364:bool, "NewVal.Reverse"=w363:bool)  [unwired: 1 in]
        n232 = Boolean To (0,1)(Boolean=w364) -> (0, 1=w360:i16)
        n233 = Boolean To (0,1)(Boolean=w363) -> (0, 1=w362:i16)
        n234 = Negate(x=w362) -> (-x=w361:i16)
        n235 = Add(x=w360, y=w361) -> (x+y=w359:i16)
        n236 = call <vilib>:"NT Write Number.vi"("Numeric"=w359, "Name"=w358) -> ()  [unwired: 9 in, 1 out]
      }
      event "Test Ring": Value Change {
        n237 = event-data() -> ("NewVal"=w368:u16)  [unwired: 1 in]
        n238 = property on="Test Ring" class="Ring (strict)"() -> ("Strings []"=w369:string[])  [unwired: 2 in, 2 out]
        n239 = Index Array(array=w369, index=w368) -> (element=w367:string)
        n240 = call <vilib>:"NT Write String.vi"("String"=w367, "Name"=w366) -> ()  [unwired: 9 in, 1 out]
      }
      event "Rec Mode": Value Change {
        # "Update globals for recording mode and path to read log from.\nClear when logging and let NetworkTables set path for vision to\nuse."
        n241 = event-data() -> ("NewVal"=w379:enum32{"Stop", "Record", "Playback"})  [unwired: 1 in]
        n242 = global write "WPI_DashboardLogging Global.vi" "Logging Filename"(path "") -> ()
        n243 = case shown="\"Stop\", \"Record\"" w379 {
          tunnel: w378 -> [_ w381 w389]
          tunnel: [_ _ w388] -> w375
          tunnel: [_ _ w387] -> _
          tunnel: w373 -> [_ _ w385]
          tunnel: cluster{i32, i32} {-250, 170} -> [_ _ w384]
          tunnel: [_ _ T18 {"Image Size"=TRUE, "Image Type"=TRUE, "Pixel Value"=TRUE, "ROI Information"=TRUE, "Zoom Factor"=FALSE} ("Image Information Shown:All Elements")] -> w371
          tunnel: [_ _ TRUE ("Zoom Factor")] -> w370
          frame Default {
          }
          frame "Stop", "Record" {
            # "Place Window too"
            n244 = invoke class="VI" method="FP.Close"(reference=w381) -> (reference out=w380:refnum<vi>)  [unwired: 2 in, 2 out]
            n245 = invoke class="VI" method="Abort VI"(reference=w380) -> ()  [unwired: 2 in, 3 out]
          }
          frame "Playback" {
            n246 = call "Open Playback Panel.vi"("Offset"=w384, "DB VI Ref"=w385, "Playback in"=w389) -> ("Playback out"=w386:refnum<vi>)  [unwired: 8 in]
            n247 = register-events(w386) -> (reference out=w388:refnum<event-registration>, error out=w387:errorcluster)  [unwired: 2 in]
          }
        }
        n248 = global write "WPI_DashboardLogging Global.vi" "Recording"(w379) -> ()
        n249 = property on="Camera Image" class="ImageControl"("Image Information Shown"=w371, "Image Information Visible"=w370) -> ()  [unwired: 2 in, 2 out]
        n250 = call <vilib>:"WPI_DashboardNT Log FieldName Cache.vi"("Operation"=enum16{"Lookup/Add", "Index", "Clear"}."Clear") -> ()  [unwired: 8 in, 3 out]
      }
      event Panel Close {
        w390 = enum32{"Stop", "Record", "Playback"}."Stop" ("Rec Mode")
        n251 = event-data() -> ()  [unwired: 1 in, 4 out]
        n252 = local write "Rec Mode"(w390) -> ()
        n253 = global write "WPI_DashboardLogging Global.vi" "Recording"(w390) -> ()
      }
      event Panel Close {
        # "Abort playback window and ourself"
        n254 = event-data() -> ()  [unwired: 1 in, 4 out]
        n255 = invoke class="VI" method="FP.Close"(reference=w395) -> (reference out=w394:refnum<vi>)  [unwired: 2 in, 2 out]
        n256 = invoke class="VI" method="Abort VI"(reference=w394) -> (error out=w393:errorcluster)  [unwired: 2 in, 2 out]
        n257 = invoke class="VI" method="Abort VI"(error in=w393) -> ()  [unwired: 2 in, 3 out]
      }
    }
  }
  n258 = property on="On/Off" class="Bool (strict)"("Visible"=w25) -> ()  [unwired: 2 in, 2 out]
  n259 = property on="Motor" class="Clust (strict)"("Visible"=w25) -> ()  [unwired: 2 in, 2 out]
  n260 = property on="Progress" class="Clust (strict)"("Visible"=w25) -> ()  [unwired: 2 in, 2 out]
  n261 = property on="Test Ring" class="Ring (strict)"("Visible"=w25) -> ()  [unwired: 2 in, 2 out]
  n262 = property on="Rev/Fwd" class="Clust (strict)"("Visible"=w25) -> ()  [unwired: 2 in, 2 out]
  n263 = property on="Camera Settings" class="Clust (strict)"("Visible"=w25) -> ()  [unwired: 2 in, 2 out]
  n264 = local write "DB Camera Config"(w25) -> ()
  n265 = global write "WPI_DashboardLogging Global.vi" "Recording"(w8) -> ()
  n266 = local write "Rec Mode"(w8) -> ()
